vi "testSendCmdFromClient.vi"(8 "error in (no error)":errorcluster) -> (0 "error out":errorcluster)   [LabVIEW 2018]
doc: "This VI sends commands from TCP client to TCP server, and receives the Ack from TCP server."
uses:
  <vilib>/addons/_JKI Toolkits/Caraya/classes/Assert/Assert Equal Value_Variant.vi
  src/TcpServer/TcpServer.lvclass
  <vilib>/addons/_JKI Toolkits/Caraya/classes/Test/Test.lvclass
  <vilib>/addons/_JKI Toolkits/Caraya/classes/Assert/Assert.lvclass
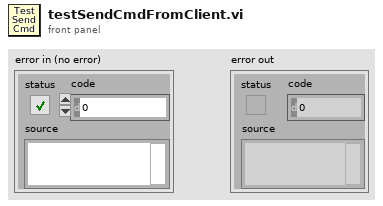
[diagram p1: front panel]
types:
  T1 = cluster{"CmdRead":refnum<user-event>, "EvtRead":refnum<user-event>, "GenRead":refnum<user-event>}
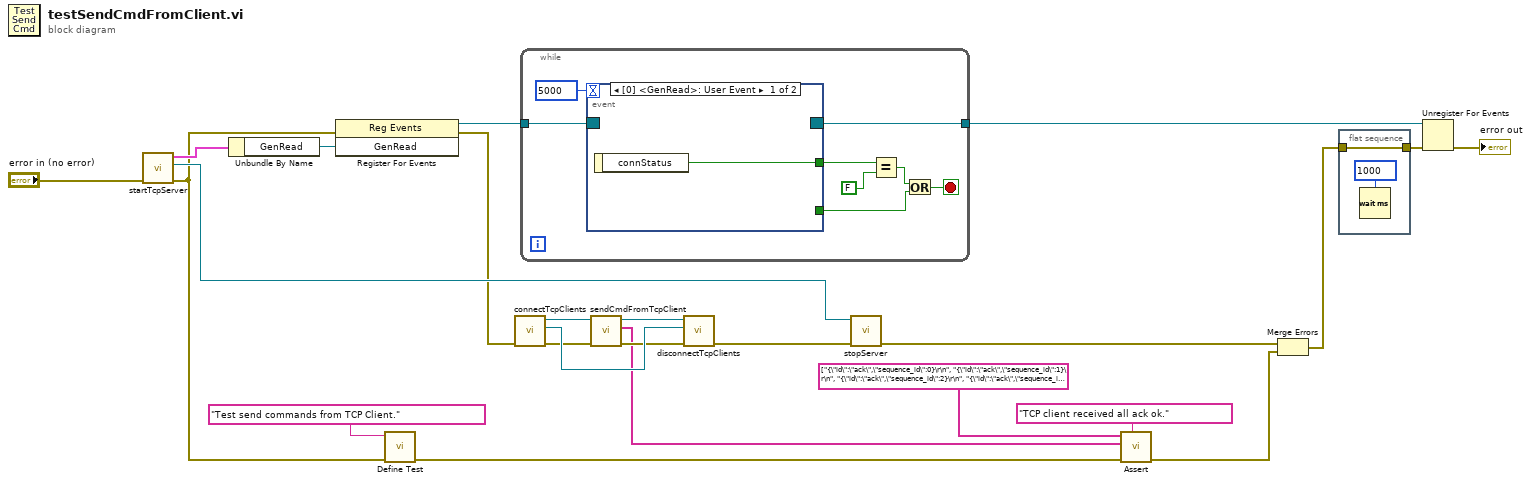
[diagram p0: block diagram]
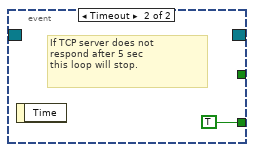
[diagram p2: hidden frame]
diagram:
  n1 = call "startTcpServer.vi"("error in (no error)"="error in (no error)") -> ("error out"=w4:errorcluster, "TcpServer out"=w11:refnum<class "TcpServer.lvclass">, "UserEvents"=w18:T1)  [unwired: 8 in]
  n2 = Unbundle By Name(w18) -> ("GenRead"=w17:refnum<user-event>)
  n3 = register-events(error in=w4, w17) -> (reference out=w24:refnum<event-registration>, error out=w3:errorcluster)  [unwired: 1 in]
  n4 = call <vilib>:"Define Test.vi"("error in (no error)"=w4, "Label (VI Title)"="Test send commands from TCP Client.") -> ("error out"=w13:errorcluster)  [unwired: 9 in]
  n5 = call "connectTcpClients.vi"("error in (no error)"=w3) -> ("error out"=w6:errorcluster, "tel connection ID out"=w15:refnum<k5>, "cmd connection ID out"=w8:refnum<k5>)  [unwired: 8 in]
  n6 = while {
    tunnel: w24 -> [w32]
    tunnel: [w31] -> w23
    stop <- w28 stop-if-true
    n7 = event shown="[0] <GenRead>: User Event" {
      selector: w32 -> [_ _]
      dyn-events: [_ _] -> w31
      timeout: 5000 -> [_ _]
      tunnel: [w33 _] -> w30
      tunnel: [_ TRUE] -> w26
      event User Event {
        n8 = event-data() -> ("connStatus"=w33:bool)  [unwired: 1 in]
      }
      event Timeout {
        # "If TCP server does not\nrespond after 5 sec\nthis loop will stop."
        n9 = event-data() -> ()  [unwired: 1 in, 1 out]
      }
    }
    n10 = Equal?(x=w30, y=FALSE) -> (x = y?=w27:bool)
    n11 = Or(x=w27, y=w26) -> (x .or. y?=w28:bool)
  }
  n12 = call "sendCmdFromTcpClient.vi"("error in (no error)"=w6, "connection ID in"=w8) -> ("error out"=w5:errorcluster, "ack received"=w1:string[], "connection ID out"=w7:refnum<k5>)  [unwired: 7 in]
  n13 = call "disconnectTcpClients.vi"("error in (no error)"=w5, "tel connection ID in"=w15, "cmd connection ID in"=w7) -> ("error out"=w20:errorcluster)  [unwired: 8 in]
  n14 = call "stopServer.vi"("error in (no error)"=w20, "tcpServer in"=w11) -> ("error out"=w21:errorcluster)  [unwired: 8 in, 1 out]
  n15 = call-poly <vilib>:"Assert.vi"("Label"="TCP client received all ack ok.", "error in (no error)"=w13, "Y"=w1, "X"=string[] ["{\"id\":\"ack\",\"sequence_id\":0}\r\n", "{\"id\":\"ack\",\"sequence_id\":1}\r\n", "{\"id\":\"ack\",\"sequence_id\":2}\r\n", "{\"id\":\"ack\",\"sequence_id\":6}\r\n", "{\"id\":\"noack\",\"sequence_id\":3}\r\n", "{\"id\":\"noack\",\"sequence_id\":4}\r\n", "{\"id\":\"noack\",\"sequence_id\":5}\r\n", "{\"id\":\"ack\",\"sequence_id\":7}\r\n", "{\"id\":\"ack\",\"sequence_id\":8}\r\n", "{\"id\":\"ack\",\"sequence_id\":9}\r\n"] ("ack received 2")) -> ("error out"=w12:errorcluster)  [unwired: 7 in]
  n16 = Merge Errors(w21, w12) -> (w9:errorcluster)
  n17 = flat-sequence {
    tunnel: w9 -> [w35]
    tunnel: [w35] -> w10
    frame #0 {
      n18 = Wait (ms)(milliseconds to wait=u32 1000) -> ()  [unwired: 1 out]
    }
  }
  n19 = Unregister For Events(event registration refnum=w23, error in=w10) -> (error out=→"error out":errorcluster)
